vi "Sebastian Espinoza Actividad 2.vi"() -> ()   [LabVIEW 2025]
uses:
  <vilib>/express/express arith-compare/Formula/XNode/ExpressFormulaBlockNode.xnode
panel:
  out "Frio":bool
  out "Caliente":bool
  out "Celsius":dbl(slide) scale=0.0..300.0
  out "Celsius":dbl
  in  "stop":bool
  out "Kelvin":dbl
  out "Fahrenheit":dbl
  out "Kelvin":dbl(slide) scale=0.0..300.0
  out "Fahrenheit":dbl(slide) scale=0.0..300.0
  in  "Temperatura (°C)":dbl(slide) scale=0.0..300.0
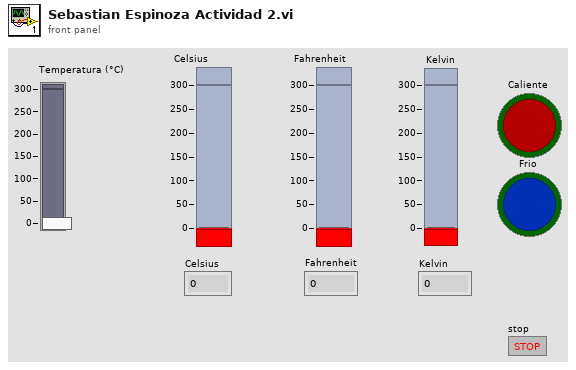
[diagram p1: front panel]
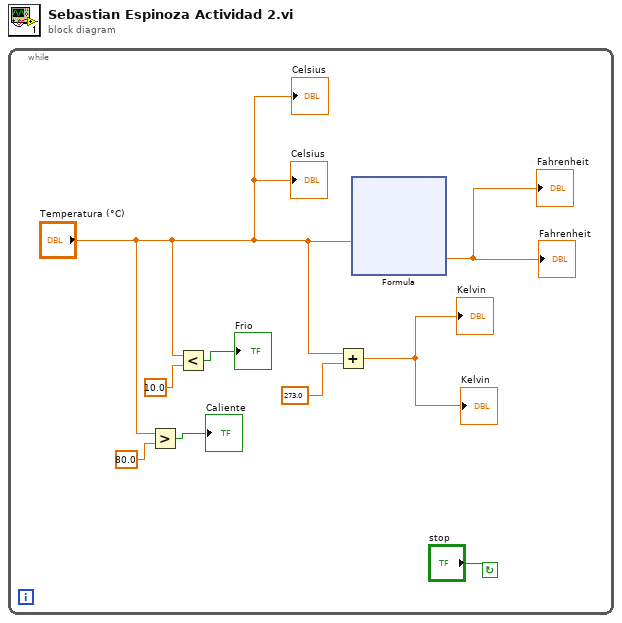
[diagram p0: block diagram]
diagram:
  n1 = while {
    stop <- "stop" continue-if-true
    n2 = Greater?(x="Temperatura (°C)", y=80.0) -> (0:→"Caliente":bool)
    n3 = Less?(x="Temperatura (°C)", y=10.0) -> (x < y?=→"Frio":bool)
    n4 = Add(x="Temperatura (°C)", y=273.0) -> (x+y=→"Kelvin" →"Kelvin":dbl)
    n5 = xnode "Formula"("X1"="Temperatura (°C)") -> ("Result"=→"Fahrenheit" →"Fahrenheit":dbl)  [unwired: 1 in, 1 out]
    "Celsius" <- "Temperatura (°C)"
    "Celsius" <- "Temperatura (°C)"
  }
